vi "Get_Set_Account_Details.vi"(0 "Updated_Account_Details":string[][](array[string]), 5 "File_Path":path, 11 "error in (no error)":errorcluster, 13 "File_Operation_Select":T1=enum."Update_Details") -> (4 "Account_Details":string[][](array[string]), 15 "error out":errorcluster)   [LabVIEW 2021]
doc: "Used to read and write the Account details form text file."
uses:
  <vilib>/Utility/file.llb/Read Delimited Spreadsheet (string).vi
  <vilib>/Utility/file.llb/Write Delimited Spreadsheet (string).vi
  Controls/File_Operation_Select.ctl
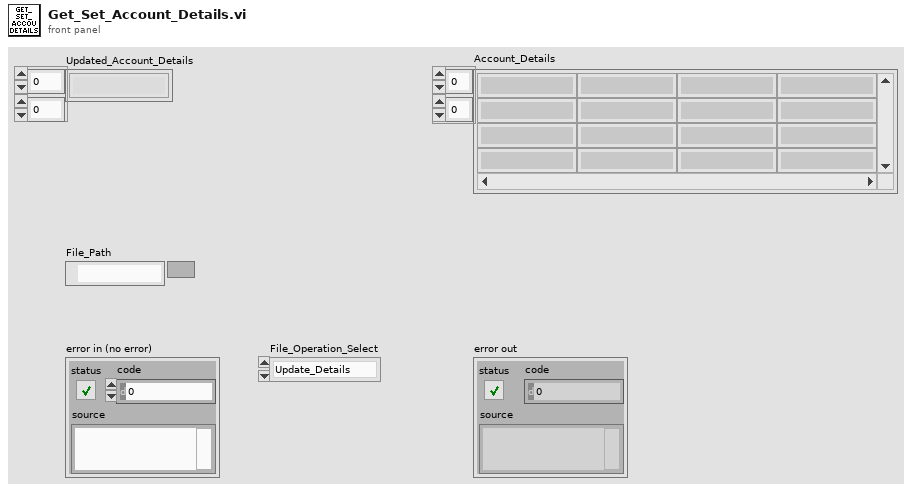
[diagram p1: front panel]
types:
  T1 = typedef "File_Operation_Select.ctl" = enum16{"Get_Details", "Update_Details"}
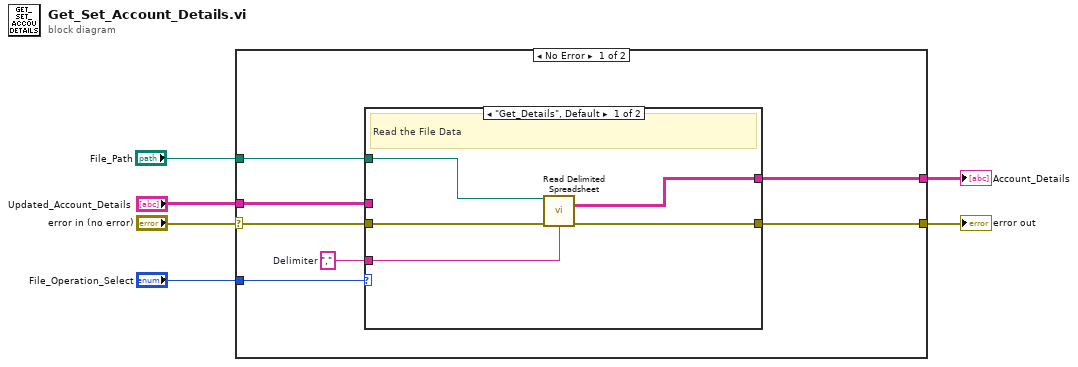
[diagram p0: block diagram]
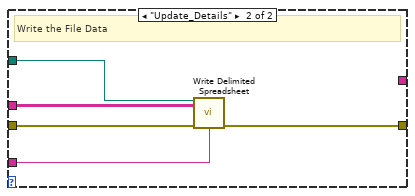
[diagram p2: hidden frame]
diagram:
  n1 = case shown="No Error" "error in (no error)" {
    selector: "error in (no error)" -> [w11 w24]
    tunnel: "File_Path" -> [w13 _]
    tunnel: [w12 w24] -> w6
    tunnel: "File_Operation_Select" -> [w10 _]
    tunnel: "Updated_Account_Details" -> [w8 _]
    tunnel: [w7 _] -> w2
    frame No Error {
      w9 = ","  # Delimiter
      n2 = case shown="\"Get_Details\", Default" w10 {
        tunnel: w13 -> [w18 w20]
        tunnel: [w17 w22] -> w12
        tunnel: w11 -> [w16 w23]
        tunnel: w9 -> [w15 w21]
        tunnel: w8 -> [_ w19]
        tunnel: [w14 _] -> w7
        frame "Get_Details", Default {
          # "Read the File Data"
          n3 = call-poly <vilib>:"Read Delimited Spreadsheet.vi"("file path (dialog if empty)"=w18, "error in (no error)"=w16, "delimiter (\\t)"=w15) -> ("all rows"=w14:string[][], "error out"=w17:errorcluster)  [unwired: 7 in, 4 out]
        }
        frame "Update_Details" {
          # "Write the File Data"
          n4 = call-poly <vilib>:"Write Delimited Spreadsheet.vi"("file path (dialog if empty)"=w20, "2D data"=w19, "error in (no error)"=w23, "delimiter (\\t)"=w21) -> ("error out"=w22:errorcluster)  [unwired: 10 in, 1 out]
        }
      }
    }
    frame Error {
    }
  }
  "error out" <- w6
  "Account_Details" <- w2
